vi "Toolkit Error Handling - Error Cluster From Error Code.vi"(4 "is warning? (False)":bool, 5 "show call chain? (False)":bool, 6 "error in":errorcluster, 8 "error message (\"\")":string, 9 "error code (0)":i32) -> (0 "error out":errorcluster)   [LabVIEW 2013]
doc: "Converts an error or warning code to an error cluster. This VI is useful when you receive a return value from a DLL call or when you return user-defined error codes."
uses:
  <vilib>/Utility/error.llb/whitespace.ctl
panel:
  in  "call chain header":string="\n<b>Complete call chain:</b>"
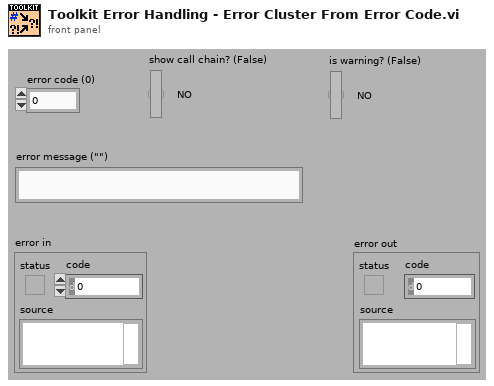
[diagram p1: front panel]
types:
  T1 = typedef "whitespace.ctl" = u16
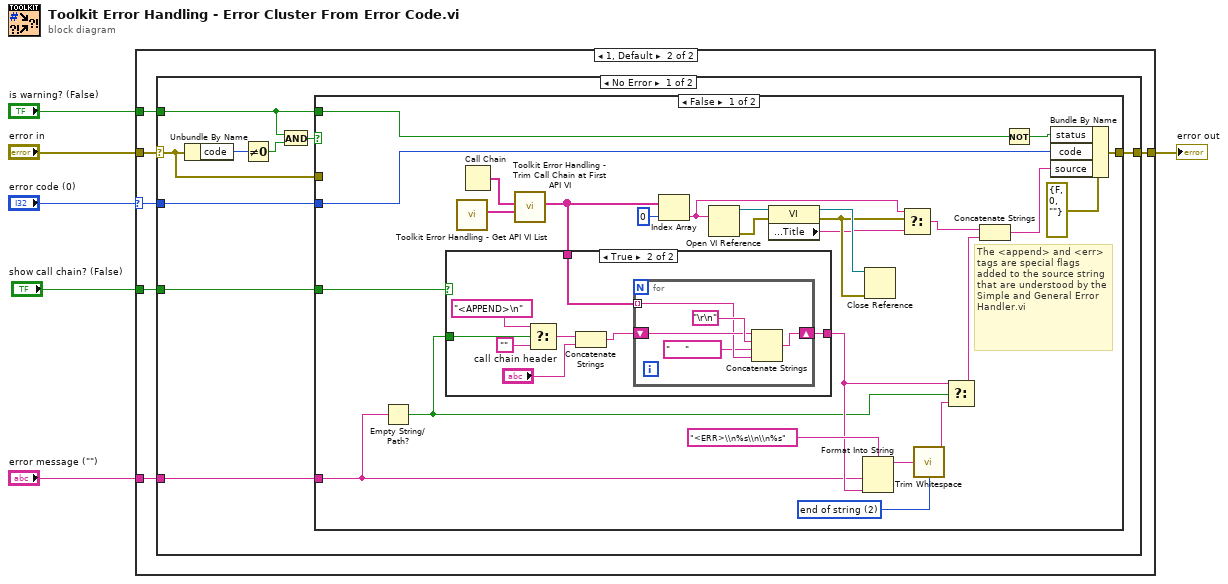
[diagram p0: block diagram]
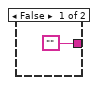
[diagram p3: hidden frame]
diagram:
  n1 = case shown="1, Default" "error code (0)" {
    selector: "error code (0)" -> [_ w11]
    tunnel: [w7 w13] -> w6
    tunnel: "error in" -> [w7 w12]
    tunnel: "error message (\"\")" -> [_ w10]
    tunnel: "is warning? (False)" -> [_ w9]
    tunnel: "show call chain? (False)" -> [_ w8]
    frame 0 {
      # "If the error code in equals zero, then propagate the error in cluster regardless of its value."
    }
    frame 1, Default {
      n2 = case shown="No Error" w12 {
        selector: w12 -> [w17 w64]
        tunnel: [w22 w64] -> w13
        tunnel: w11 -> [w21 _]
        tunnel: w10 -> [w16 _]
        tunnel: w9 -> [w15 _]
        tunnel: w8 -> [w14 _]
        frame No Error {
          n3 = Unbundle By Name(w17) -> ("code"=w20:i32)
          n4 = Not Equal To 0?(x=w20) -> (x != 0?=w18:bool)
          n5 = And(x=w15, y=w18) -> (x .and. y?=w19:bool)
          n6 = case shown="False" w19 {
            tunnel: [w48 w63] -> w22
            tunnel: w21 -> [w44 _]
            tunnel: w17 -> [_ w63]
            tunnel: w15 -> [w35 _]
            tunnel: w16 -> [w31 _]
            tunnel: w14 -> [w23 _]
            frame False {
              w27 = T1 2 items=["both", "start of string", "end of string"] ("location (both)")
              # "The <append> and <err> tags are special flags added to the source string that are understood by the Simple and General Error Handler.vi"
              n7 = Empty String/Path?(string/path=w31) -> (empty?=w30:bool)
              n8 = call "Toolkit Error Handling - Get API VI List.vi"() -> ("API VI List"=w25:string[])  [unwired: 10 in, 1 out]
              n9 = Call Chain() -> (call chain=w26:string[])
              n10 = call "Toolkit Error Handling - Trim Call Chain at First API VI.vi"("API VI List"=w25, "call chain"=w26) -> ("trimmed call chain"=w24:string[])  [unwired: 8 in, 1 out]
              n11 = case shown="True" w23 {
                tunnel: ["" w57] -> w33
                tunnel: w24 -> [_ w50]
                tunnel: w30 -> [_ w54]
                frame False {
                }
                frame True {
                  n12 = Select(t="<APPEND>\n", s=w54, f="") -> (s? t:f=w51:string)
                  n13 = Concatenate Strings(w51, "call chain header") -> (w55:string)
                  n14 = for {
                    tunnel: w50 -> [w59] mode=indexing
                    shift-right: [w62] -> w57
                    shift-left: w55 -> [w60]
                    n15 = Concatenate Strings(w60, "\r\n", "     ", w59) -> (w62:string)
                  }
                }
              }
              n16 = Index Array(array=w24, index=0) -> (element=w38:string)
              n17 = Open VI Reference(vi path=w38) -> (vi reference=w42:refnum<vi>, error out=w41:errorcluster)  [unwired: 5 in]
              n18 = property class="VI"(reference=w42, error in=w41) -> (reference out=w40:refnum<vi>, error out=w39:errorcluster, "Front Panel Window:Title"=w37:string)
              n19 = Format Into String(format string="<ERR>\\n%s\\n\\n%s", w31, w33) -> (resulting string=w29:string)  [unwired: 2 in, 1 out]
              n20 = Close Reference(reference=w40, error in (no error)=w39) -> ()  [unwired: 1 out]
              n21 = Select(t=w38, s=w39, f=w37) -> (s? t:f=w36:string)
              n22 = call <vilib>:"Trim Whitespace.vi"("string"=w29, "location (both)"=w27) -> ("trimmed string"=w28:string)
              n23 = Select(t=w33, s=w30, f=w28) -> (s? t:f=w32:string)
              n24 = Concatenate Strings(w36, w32) -> (w46:string)
              n25 = Not(x=w35) -> (.not. x?=w45:bool)
              n26 = Bundle By Name(cluster=errorcluster {"status"=FALSE, "code"=0, "source"=""} ("error out"), "status"=w45, "code"=w44, "source"=w46) -> (w48:errorcluster)
            }
            frame True {
              # "If the error code input is setting a warning, and a warning is already set on the wire, then we\ngo with the one already on the wire."
            }
          }
        }
        frame Error {
          # "An error in trumps any error code input."
        }
      }
    }
  }
  "error out" <- w6
